vi "Read Pump Value.vi"(8 "error in":errorcluster, 11 "TSI 3025 in":refnum<class "TSI 3025.lvclass">) -> (0 "error out":errorcluster, 2 "Pump Value":dbl, 3 "TSI 3025 out":refnum<class "TSI 3025.lvclass">)   [LabVIEW 2013, in "TSI 3025.lvclass"]
uses:
  TSI 3025.lvclass
  CPC.lvclass/CPC.ctl
  Accessors/Read Session Handle.vi
  Accessors/Write Session Handle.vi
  Reusable/Session APIs/Serial/Public/Get Data/Get Long Integer.vi
  Reusable/Session APIs/Serial/Serial Session.lvclass
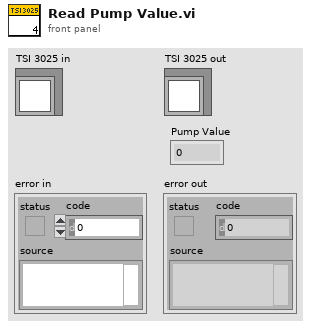
[diagram p1: front panel]
types:
  T1 = typedef "Serial Session.lvclass/Session Handle.ctl" = refnum<data-value>
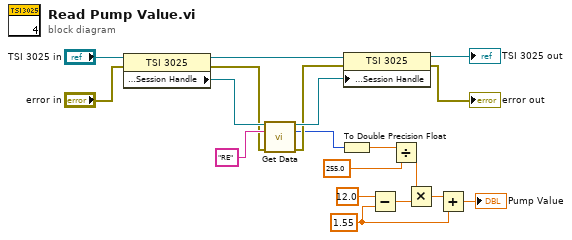
[diagram p0: block diagram]
diagram:
  w2 = 1.55 ("y")
  n1 = property class="TSI 3025"(reference="TSI 3025 in", error in="error in") -> (reference out=w16:refnum<class "TSI 3025.lvclass">, error out=w15:errorcluster, "Accessors:Session Handle"=w18:T1)
  n2 = call-poly "Get Data.vi"("Session Handle in"=w18, "CMD"="RE" ("string"), "error in"=w15) -> ("Session Handle out"=w17:T1, "DataOut"=w7:i32, "error out"=w14:errorcluster)  [unwired: 10 in]
  n3 = To Double Precision Float(number=w7) -> (double precision float=w8:dbl)
  n4 = property class="TSI 3025"(reference=w16, error in=w14, "Accessors:Session Handle"=w17) -> (reference out=→"TSI 3025 out":refnum<class "TSI 3025.lvclass">, error out=→"error out":errorcluster)
  n5 = Subtract(x=12.0, y=w2) -> (x-y=w4:dbl)
  n6 = Divide(x=w8, y=255.0) -> (x/y=w5:dbl)
  n7 = Multiply(x=w5, y=w4) -> (x*y=w3:dbl)
  n8 = Add(x=w3, y=w2) -> (x+y=→"Pump Value":dbl)
